vi "Write Message.vi"(8 "error in (no error)":errorcluster, 10 "Message":string, 11 "Test Log in":refnum<class "Test Log.lvclass">) -> (0 "error out":errorcluster, 3 "Test Log out":refnum<class "Test Log.lvclass">)   [LabVIEW 2015, in "Test Log.lvclass"]
uses:
  Test Log.lvclass
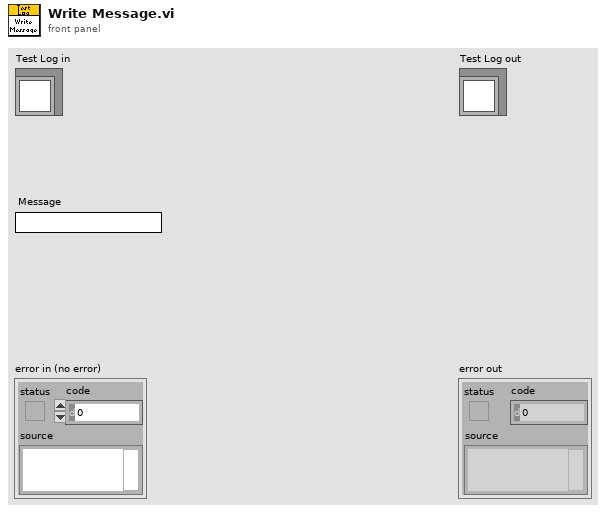
[diagram p1: front panel]
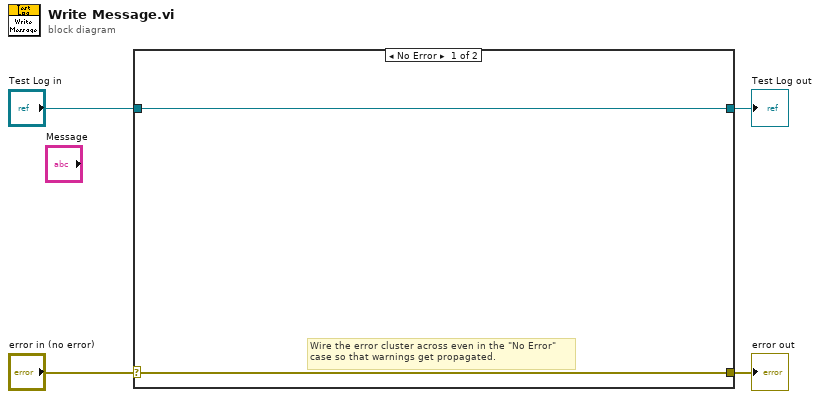
[diagram p0: block diagram]
diagram:
  n1 = case shown="No Error" "error in (no error)" {
    selector: "error in (no error)" -> [w5 w8]
    tunnel: [w5 w8] -> w3
    tunnel: [w6 w7] -> w1
    tunnel: "Test Log in" -> [w6 w7]
    frame No Error {
      # "Wire the error cluster across even in the \"No Error\"\ncase so that warnings get propagated."
    }
    frame Error {
    }
  }
  "error out" <- w3
  "Test Log out" <- w1
